vi "Temperature Analysis.vi"() -> ()   [LabVIEW 2018]
uses:
  <vilib>/Analysis/baseanly.llb/Mean (DBL).vi
  <vilib>/Analysis/NI_AALBase.lvlib
panel:
  out "Mean":dbl
  out "Min":dbl
  out "Max":dbl
  out "Temp Graph":dbl[](graph)
  out "Temperature":dbl(graph)
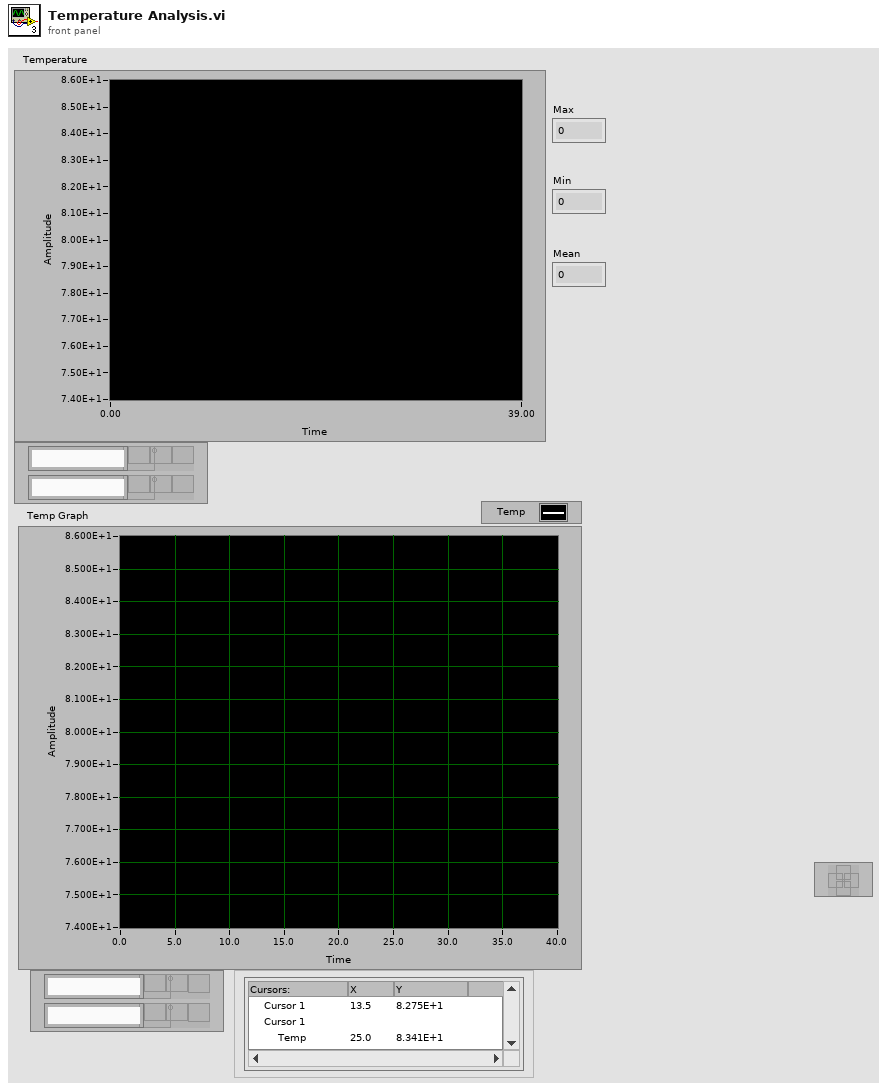
[diagram p1: front panel]
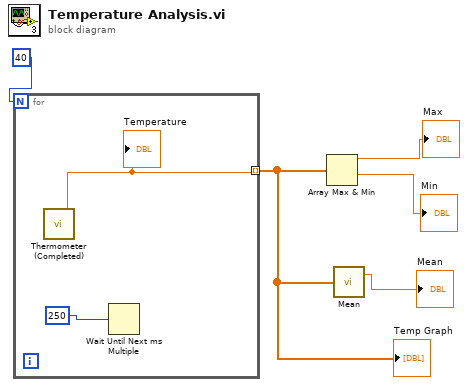
[diagram p0: block diagram]
diagram:
  n1 = for {
    N: 40 -> [_]
    tunnel: [w6] -> w4 mode=indexing
    n2 = call "Thermometer (Completed).vi"() -> ("Temperature (deg F)"=w6:dbl)  [unwired: 1 in]
    "Temperature" <- w6
    n3 = Wait Until Next ms Multiple(millisecond multiple=250) -> ()  [unwired: 1 out]
  }
  "Temp Graph" <- w4
  n4 = Array Max & Min(array=w4) -> (max value=→"Max":dbl, min value=→"Min":dbl)  [unwired: 2 out]
  n5 = call-poly <vilib>:"Mean.vi"("X"=w4) -> ("mean"=→"Mean":dbl)  [unwired: 1 out]
